vi "stop tasks.vi"(8 "error in (no error)":errorcluster, 11 "Waveform in":refnum<class "Waveform.lvclass">) -> (0 "error out":errorcluster, 3 "Waveform out":refnum<class "Waveform.lvclass">)   [LabVIEW 2012, in "Waveform.lvclass"]
uses:
  Waveform.lvclass
  Waveform.lvclass/Waveform.ctl
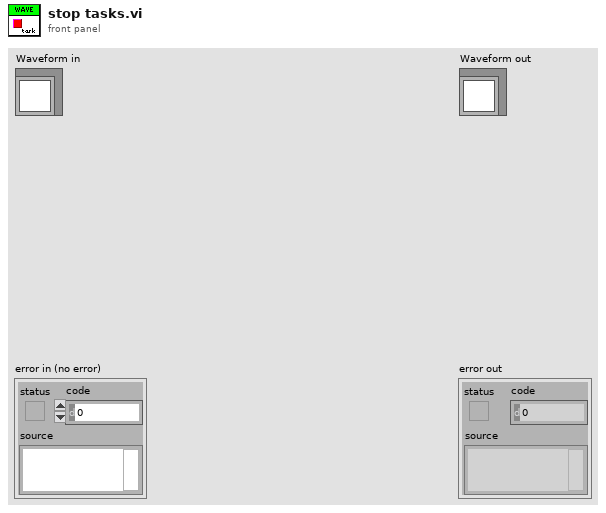
[diagram p1: front panel]
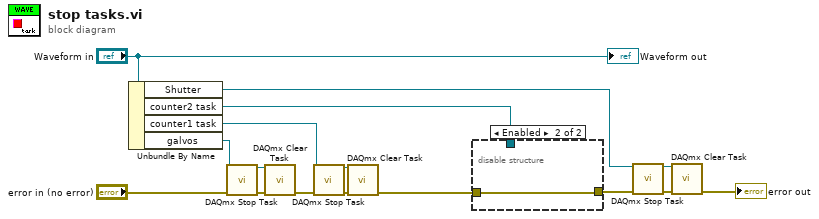
[diagram p0: block diagram]
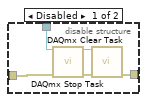
[diagram p2: hidden frame]
diagram:
  n1 = Unbundle By Name("Waveform in") -> ("Shutter"=w3:refnum<k21>, "counter2 task"=w8:refnum<k21>, "counter1 task"=w9:refnum<k21>, "galvos"=w10:refnum<k21>)
  n2 = call <vilib>:"DAQmx Stop Task.vi"("task/channels in"=w10, "error in"="error in (no error)") -> ("task out"=w12:refnum<k21>, "error out"=w13:errorcluster)  [unwired: 12 in]
  n3 = call <vilib>:"DAQmx Clear Task.vi"("task in"=w12, "error in"=w13) -> ("error out"=w7:errorcluster)  [unwired: 13 in]
  n4 = call <vilib>:"DAQmx Stop Task.vi"("task/channels in"=w9, "error in"=w7) -> ("task out"=w11:refnum<k21>, "error out"=w14:errorcluster)  [unwired: 12 in]
  n5 = call <vilib>:"DAQmx Clear Task.vi"("task in"=w11, "error in"=w14) -> ("error out"=w1:errorcluster)  [unwired: 13 in]
  n6 = disable-structure shown="Enabled" {
    disable-tunnel: w8 -> [w19 _]
    disable-tunnel: [w18 w22] -> w5
    disable-tunnel: w1 -> [w17 w22]
    frame Disabled {
      n7 = call <vilib>:"DAQmx Stop Task.vi"("task/channels in"=w19, "error in"=w17) -> ("task out"=w21:refnum<k21>, "error out"=w20:errorcluster)  [unwired: 12 in]
      n8 = call <vilib>:"DAQmx Clear Task.vi"("task in"=w21, "error in"=w20) -> ("error out"=w18:errorcluster)  [unwired: 13 in]
    }
    frame Enabled {
    }
  }
  n9 = call <vilib>:"DAQmx Stop Task.vi"("task/channels in"=w3, "error in"=w5) -> ("task out"=w2:refnum<k21>, "error out"=w6:errorcluster)  [unwired: 12 in]
  n10 = call <vilib>:"DAQmx Clear Task.vi"("task in"=w2, "error in"=w6) -> ("error out"=→"error out":errorcluster)  [unwired: 13 in]
  "Waveform out" <- "Waveform in"
